vi "Update References.vi"(8 "error in":errorcluster, 10 "Cluster":T1) -> (0 "error out":errorcluster)   [LabVIEW 2024, in "GUI.lvlib"]
doc: "updating reference to all modules\n\n_____\nCreated using DQMH Framework: Event Scripter 7.1.0.1503."
uses:
  GUI.lvlib
  GUI data ref.ctl
  Update References Argument--cluster.ctl
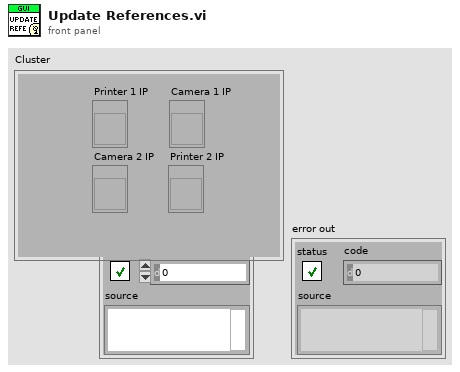
[diagram p1: front panel]
types:
  T1 = typedef "GUI data ref.ctl" = cluster{"Printer 1 IP":refnum<vi>, "Camera 2 IP":refnum<vi>, "Camera 1 IP":refnum<vi>, "Printer 2 IP":refnum<vi>}
  T2 = typedef "GUI.lvlib/Update References Argument--cluster.ctl" = cluster{"Cluster":T1}
  T3 = typedef "GUI.lvlib/Broadcast Events--cluster.ctl" = cluster{"Module Did Init":refnum<user-event>, "Status Updated":refnum<user-event>, "Error Reported":refnum<user-event>, "Module Did Stop":refnum<user-event>, "Update Module Execution Status":refnum<user-event>, "Update References":refnum<user-event>}
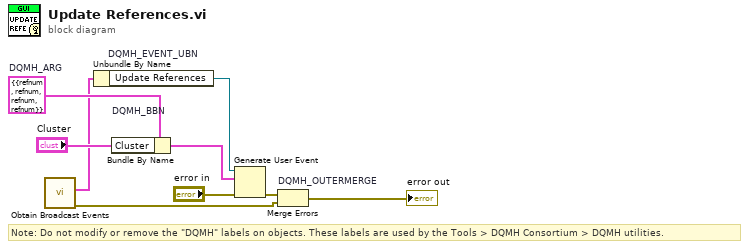
[diagram p0: block diagram]
diagram:
  w4 = T2 {"Cluster"={"Printer 1 IP"=refnum, "Camera 2 IP"=refnum, "Camera 1 IP"=refnum, "Printer 2 IP"=refnum}}  # DQMH_ARG
  # "Note: Do not modify or remove the \"DQMH\" labels on objects. These labels are used by the Tools > DQMH Consortium > DQMH utilities."
  n1 = call "Obtain Broadcast Events.vi"() -> ("error out"=w2:errorcluster, "GUI Broadcast Events"=w1:T3)  [unwired: 10 in]
  n2 = Unbundle By Name "DQMH_EVENT_UBN"(w1) -> ("Update References"=w6:refnum<user-event>)
  n3 = Bundle By Name "DQMH_BBN"(cluster=w4, "Cluster"="Cluster") -> (w7:T2)
  n4 = Generate User Event(user event=w6, event data cluster=w7, error in="error in") -> (error out=w5:errorcluster)  [unwired: 1 in, 1 out]
  n5 = Merge Errors "DQMH_OUTERMERGE"(w5, w2) -> (→"error out":errorcluster)
